vi "Find VI (In Project Item).vi"(10 "VI Name":string, 11 "ProjectItem in":refnum<vi>) -> (1 "Found?":bool, 2 "VI ProjectItem Refnum":refnum<vi>, 3 "ProjectItem out":refnum<vi>)   [LabVIEW 2019, in "QControl Creation.lvclass"]
doc: "<b> </b> <b> </b>\n©2016 Q Software Innovations, LLC (QSI)\nwritten by Quentin Alldredge\nproduced in LabVIEW 2015\n\nsupport@qsoftwareinnovations.com\nwww.qsoftwareinnovations.com\n\nAll rights reserved.\n\nRedistribution and use in source and binary forms, with or without modification, are permitted provided that the following conditions are met:\n\n * Redistributions of source code must retain the above copyright notice, this list of conditions and the following disclaimer.\n * Redistributions in binary form must reproduce the above copyright notice, this list of conditions and the following disclaimer in the documentation and/or other materials provided with the distribution.\n * Neither the name of Q Software Innovations, LLC. nor the names of its contributors may be used to endorse or promote products derived from this software without specific prior written permission.\n\nTHIS SOFTWARE IS PROVIDED BY THE COPYRIGHT HOLDERS AND CONTRIBUTORS \"AS IS\" AND ANY EXPRESS OR IMPLIED WARRANTIES, INCLUDING, BUT NOT LIMITED TO, THE IMPLIED WARRANTIES OF MERCHANTABILITY AND FITNESS FOR A PARTICULAR PURPOSE ARE DISCLAIMED. IN NO EVENT SHALL THE COPYRIGHT OWNER OR CONTRIBUTORS BE LIABLE FOR ANY DIRECT, INDIRECT, INCIDENTAL, SPECIAL, EXEMPLARY, OR CONSEQUENTIAL DAMAGES (INCLUDING, BUT NOT LIMITED TO, PROCUREMENT OF SUBSTITUTE GOODS OR SERVICES; LOSS OF USE, DATA, OR PROFITS; OR BUSINESS INTERRUPTION) HOWEVER CAUSED AND ON ANY THEORY OF LIABILITY, WHETHER IN CONTRACT, STRICT LIABILITY, OR TORT (INCLUDING NEGLIGENCE OR OTHERWISE) ARISING IN ANY WAY OUT OF THE USE OF THIS SOFTWARE, EVEN IF ADVISED OF THE POSSIBILITY OF SUCH DAMAGE."
uses:
  QControl Creation.lvclass
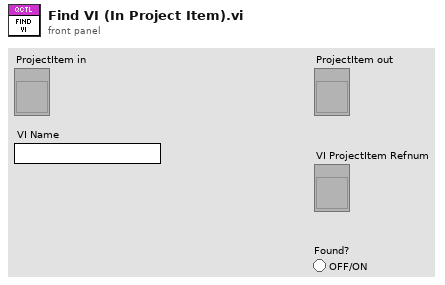
[diagram p1: front panel]
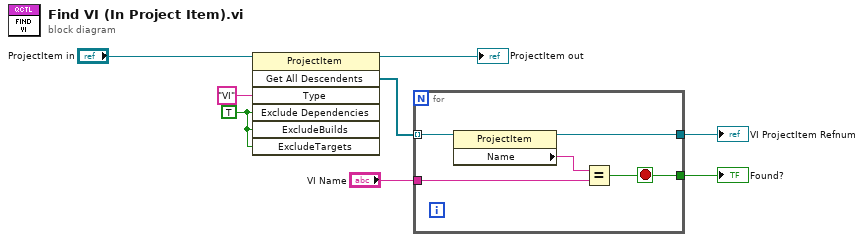
[diagram p0: block diagram]
diagram:
  w8 = TRUE ("ExcludeDependencies")
  n1 = invoke class="ProjectItem" method="Get All Descendents"(reference="ProjectItem in", "Type"="VI", "Exclude Dependencies"=w8, "ExcludeBuilds"=w8, "ExcludeTargets"=w8) -> (reference out=→"ProjectItem out":refnum<vi>, "All Descendents"=w6:refnum<vi>[])  [unwired: 2 in, 5 out]
  n2 = for {
    tunnel: w6 -> [w13] mode=indexing
    tunnel: "VI Name" -> [w11]
    tunnel: [w10] -> w3
    tunnel: [w9] -> w4
    stop <- w9 stop-if-true
    n3 = property class="ProjectItem"(reference=w13) -> (reference out=w10:refnum<vi>, "Name"=w12:string)  [unwired: 1 in, 1 out]
    n4 = Equal?(x=w12, y=w11) -> (x = y?=w9:bool)
  }
  "Found?" <- w4
  "VI ProjectItem Refnum" <- w3
